vi "Get Path and Working Directory.vi"(8 "error in":errorcluster, 10 "Element to show log for":string, 11 "VI in":refnum<vi>) -> (0 "error out":errorcluster, 2 "/path value":string, 3 "Working Directory":path)   [LabVIEW 2018, in "TortoiseGit Show Log.lvlib"]
uses:
  TortoiseGit Show Log.lvlib
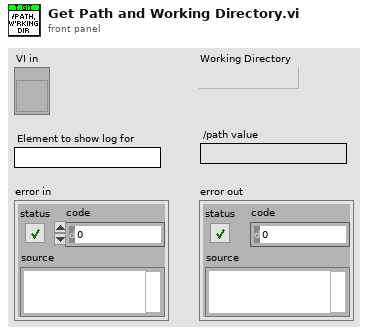
[diagram p1: front panel]
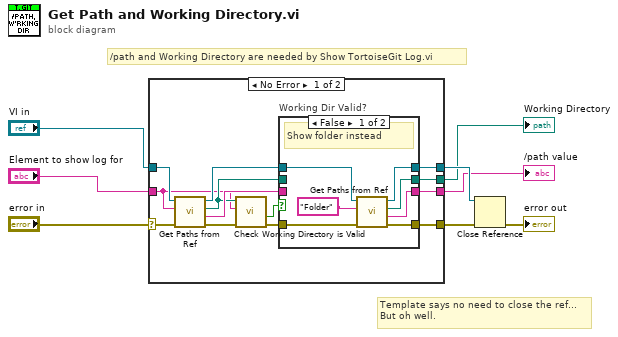
[diagram p0: block diagram]
diagram:
  # "Template says no need to close the ref...\nBut oh well."
  # "/path and Working Directory are needed by Show TortoiseGit Log.vi"
  n1 = case shown="No Error" "error in" {
    selector: "error in" -> [w20 w34]
    tunnel: "VI in" -> [w21 w33]
    tunnel: [w10 w34] -> w5
    tunnel: [w11 w33] -> w6
    tunnel: "Element to show log for" -> [w9 _]
    tunnel: [w15 _] -> w2
    tunnel: [w12 _] -> w1
    frame No Error {
      n2 = call "Get Paths from Ref.vi"("error in"=w20, "Element to show log for"=w9, "VI in"=w21) -> ("error out"=w19:errorcluster, "/path"=w14:string, "Working Directory"=w13:path, "VI out"=w17:refnum<vi>)  [unwired: 5 in]
      n3 = call "Check Working Directory is Valid.vi"("error in"=w19, "Element to show log for"=w9, "Working directory"=w13) -> ("error out"=w16:errorcluster, "Valid?"=w18:bool)  [unwired: 7 in]
      n4 = case "Working Dir Valid?" shown="False" w18 {
        tunnel: w17 -> [w26 w29]
        tunnel: [w28 w30] -> w10
        tunnel: w16 -> [w27 w30]
        tunnel: [w25 w32] -> w15
        tunnel: w14 -> [_ w32]
        tunnel: w13 -> [_ w31]
        tunnel: [w23 w31] -> w12
        tunnel: [w24 w29] -> w11
        frame False {
          # "Show folder instead"
          n5 = call "Get Paths from Ref.vi"("error in"=w27, "Element to show log for"="Folder", "VI in"=w26) -> ("error out"=w28:errorcluster, "/path"=w25:string, "Working Directory"=w23:path, "VI out"=w24:refnum<vi>)  [unwired: 5 in]
        }
        frame True {
          # "We already have paths"
        }
      }
    }
    frame Error {
    }
  }
  "Working Directory" <- w1
  "/path value" <- w2
  n6 = Close Reference(reference=w6, error in (no error)=w5) -> (error out=→"error out":errorcluster)
